vi "periodicity property.vi"() -> ()   [LabVIEW 2014]
panel:
  out "Array":cdb[](array[numeric]) format="%#.3f"
  in  "N2":dbl=4.0 format="%#_13g"
  in  "N":dbl=4.0 format="%#_13g"
  out "Array 2":cdb[](array[numeric]) format="%#.3f"
  out "Waveform Chart 2":dbl[][](graph)
  in  "stop 2":bool
  in  "stop":bool
  out "Waveform Chart":dbl[][](graph)
  # "PERIODICITY PROPERTY"
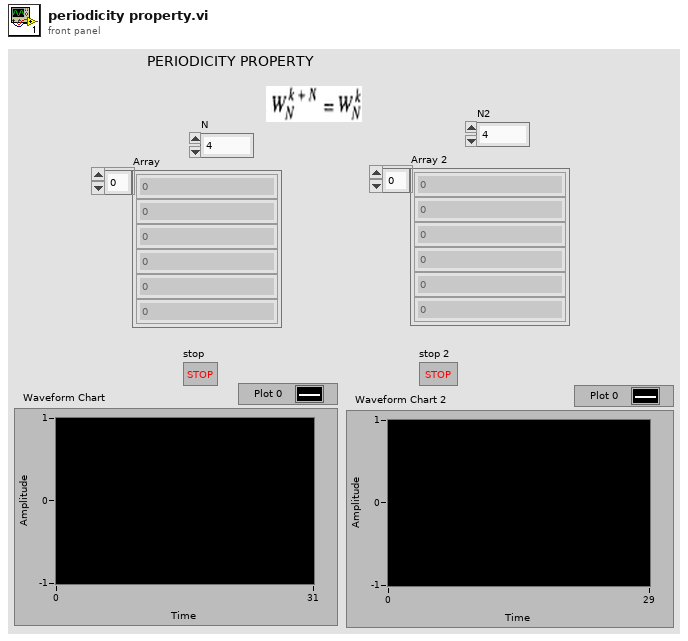
[diagram p1: front panel]
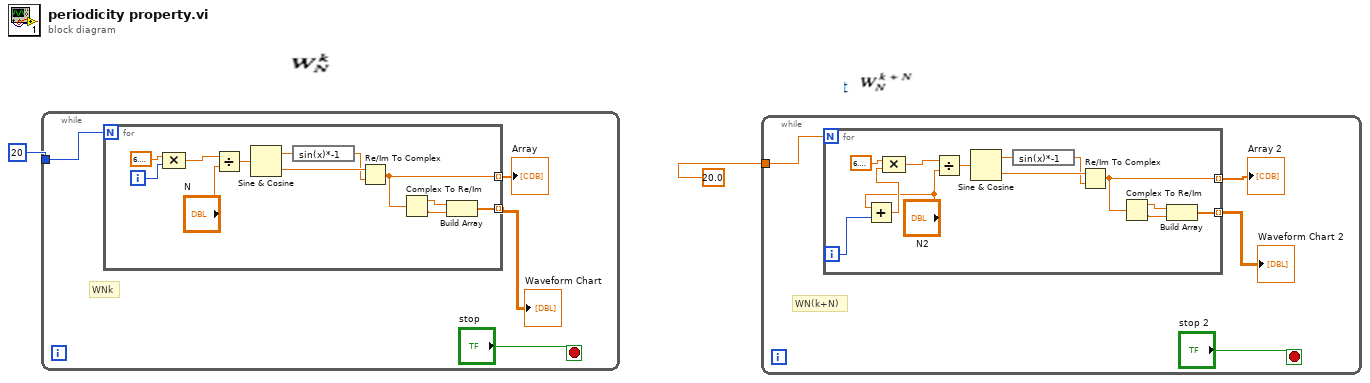
[diagram p0: block diagram]
diagram:
  n1 = while {
    tunnel: 20 -> [w6]
    stop <- "stop" stop-if-true
    # "WNk"
    n2 = for {
      N: w6 -> [_]
      tunnel: [w8] -> w4 mode=indexing
      tunnel: [w7] -> w3 mode=indexing
      i -> [w18]
      n3 = Compound Arithmetic op=MULTIPLY(6.283185307179586, w18) -> (w16:dbl)
      n4 = Divide(x=w16, y="N") -> (x/y=w14:dbl)
      n5 = Sine & Cosine(0:w14) -> (1:w12:dbl, 2:w13:dbl)
      n6 = expression code="sin(x)*-1"(w12) -> (w11:dbl)
      n7 = Re/Im To Complex(1:w11, 2:w13) -> (0:w7:cdb)
      n8 = Complex To Re/Im(x + iy=w7) -> (x=w10:dbl, y=w9:dbl)
      n9 = Build Array(w10, w9) -> (w8:dbl[])
    }
    "Waveform Chart" <- w4
    "Array" <- w3
  }
  n10 = while {
    tunnel: 20.0 ("Numeric 2") -> [w22]
    stop <- "stop 2" stop-if-true
    # "WN(k+N)"
    n11 = for {
      N: w22 -> [_]
      tunnel: [w27] -> w20 mode=indexing
      tunnel: [w24] -> w19 mode=indexing
      i -> [w25]
      n12 = Add(x="N2", y=w25) -> (x+y=w26:dbl)
      n13 = Compound Arithmetic op=MULTIPLY(6.283185307179586, w26) -> (w34:dbl)
      n14 = Divide(x=w34, y="N2") -> (x/y=w33:dbl)
      n15 = Sine & Cosine(0:w33) -> (1:w31:dbl, 2:w32:dbl)
      n16 = expression code="sin(x)*-1"(w31) -> (w30:dbl)
      n17 = Re/Im To Complex(1:w30, 2:w32) -> (0:w24:cdb)
      n18 = Complex To Re/Im(x + iy=w24) -> (x=w29:dbl, y=w28:dbl)
      n19 = Build Array(w29, w28) -> (w27:dbl[])
    }
    "Waveform Chart 2" <- w20
    "Array 2" <- w19
  }
